vi "CH_LM App DAQ Dispatcher.vi"(4 "DAQ Command":T2={"Wait at Rendesvouz"=FALSE, "Command"="", "Sample Collection"=enum."Continuous", "Sample Size"=100, "Collection Mode"=enum."Streaming", "T / ms"=1.0, "NofBins"=7, "Point(s)"=1, "Log Data File"=path "", "Log data to File"=FALSE, "Pause"=FALSE, "Meter Index"=0, "Data format"=0, "Delivery Mode"=enum."Last", "Start/Stop Button"=refnum, "Point(s) Array"=[]} {"Point(s) Array" min=1 max=20000; "Point(s)" min=1 max=20000; "Sample Size" min=1}, 5 "Rendezvous":T4, 6 "error in (no error)":errorcluster, 8 "Devices":T1[](array[typedef]) {"Probe Diameter" format="%#.2g"}, 9 "Parent ref":refnum<vi>) -> (0 "error out":errorcluster, 2 "timed out":bool)   [LabVIEW 2012, in "CH_LM App.lvlib"]
doc: "This VI is used to dispatch new DAQ threads."
uses:
  CH_LM App.lvlib
  _CH_LM/CH_LM FGV Functions.ctl
  CH_LM.lvlib
  CH_LM App DAQ Command.ctl
  CH_LM App DeviceListElement.ctl
  CH_LM/CH_LM Measurement Delivery Mode.ctl
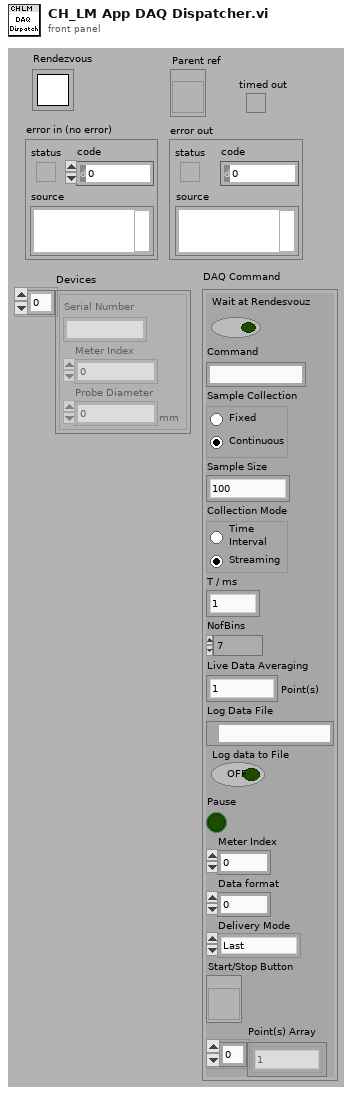
[diagram p1: front panel]
types:
  T1 = typedef "CH_LM App.lvlib/CH_LM App DeviceListElement.ctl" = cluster{"Serial Number":string, "Meter Index":i32, "Probe Diameter":dbl[unit]}
  T2 = typedef "CH_LM App.lvlib/CH_LM App DAQ Command.ctl" = cluster{"Wait at Rendesvouz":bool, "Command":string, "Sample Collection":enum32{"Fixed", "Continuous"}, "Sample Size":i32, "Collection Mode":enum32{"Time\nInterval", "Streaming"}, "T / ms":dbl, "NofBins":i32, "Point(s)":u32, "Log Data File":path, "Log data to File":bool, "Pause":bool, "Meter Index":i32, "Data format":u16, "Delivery Mode":T3, "Start/Stop Button":refnum<vi>, "Point(s) Array":u32[]}
  T3 = typedef "CH_LM.lvlib/CH_LM Measurement Delivery Mode.ctl" = enum16{"Last", "Stream"}
  T4 = typedef "Rendezvous RefNum" = refnum<k1>
  T5 = typedef "CH_LM.lvlib/CH_LM FGV Functions.ctl" = enum16{"create", "get", "set", "remove", "clear", "getBySerial"}
  T6 = enum32{"Invalid", "Standard", "Closed", "Hidden", "Minimized", "Maximized"}
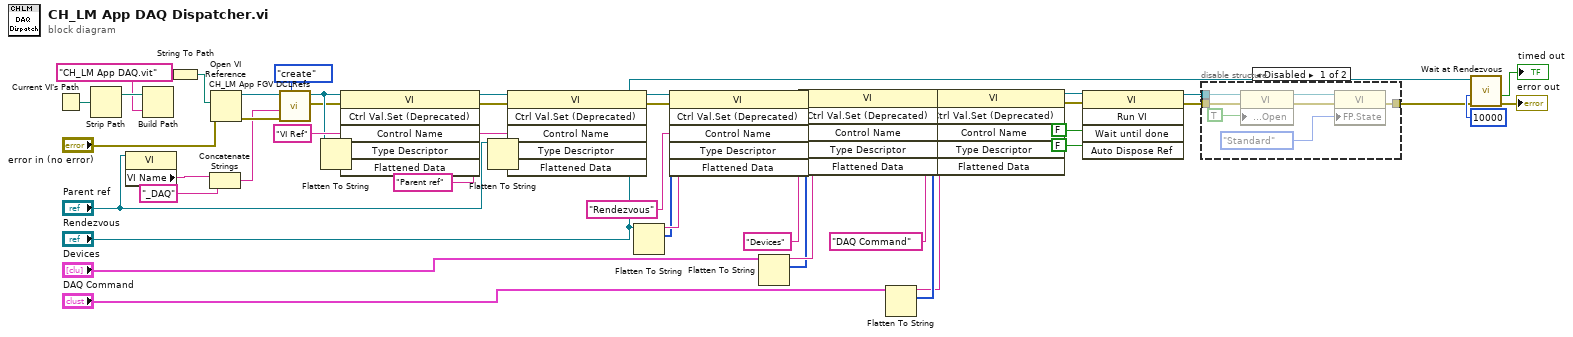
[diagram p0: block diagram]
diagram:
  w2 = "CH_LM App DAQ.vit"
  n1 = Current VI's Path() -> (path=w50:path)
  n2 = Strip Path(path=w50) -> (stripped path=w49:path)  [unwired: 1 out]
  n3 = property class="VI"(reference="Parent ref") -> ("VI Name"=w11:string)  [unwired: 1 in, 2 out]
  n4 = Build Path(base path=w49, name or relative path=w2) -> ()  [unwired: 1 out]
  n5 = String To Path(string=w2) -> (path=w3:path)
  n6 = Concatenate Strings(w11, "_DAQ" ("string")) -> (w9:string)
  n7 = Open VI Reference(vi path=w3, error in (no error)="error in (no error)") -> (vi reference=w34:refnum<vi>, error out=w33:errorcluster)  [unwired: 4 out]
  n8 = call "CH_LM App FGV DCLRefs.vi"("Function"=CH_LM_FGV_Functions."create", "error in (no error)"=w33, "VI Name"=w9, "VI Ref"=w34) -> ("error out"=w30:errorcluster, "VI Ref"=w31:refnum<vi>)  [unwired: 6 out]
  n9 = Flatten To String(anything=w31) -> (data string=w44:string, type string=w45:i16[])  [unwired: 1 in, 3 out]
  n10 = invoke class="VI" method="Ctrl Val.Set (Deprecated)"(reference=w31, error in=w30, "Control Name"="VI Ref", "Type Descriptor"=w45, "Flattened Data"=w44) -> (reference out=w26:refnum<vi>, error out=w23:errorcluster)  [unwired: 1 in, 4 out]
  n11 = Flatten To String(anything="Parent ref") -> (data string=w29:string, type string=w28:i16[])  [unwired: 1 in, 3 out]
  n12 = invoke class="VI" method="Ctrl Val.Set (Deprecated)"(reference=w26, error in=w23, "Control Name"="Parent ref", "Type Descriptor"=w28, "Flattened Data"=w29) -> (reference out=w25:refnum<vi>, error out=w24:errorcluster)  [unwired: 1 in, 4 out]
  n13 = Flatten To String(anything="Rendezvous") -> (data string=w41:string, type string=w40:i16[])  [unwired: 1 in, 3 out]
  n14 = invoke class="VI" method="Ctrl Val.Set (Deprecated)"(reference=w25, error in=w24, "Control Name"="Rendezvous", "Type Descriptor"=w40, "Flattened Data"=w41) -> (reference out=w14:refnum<vi>, error out=w13:errorcluster)  [unwired: 1 in, 4 out]
  n15 = Flatten To String(anything="Devices") -> (data string=w37:string, type string=w36:i16[])  [unwired: 1 in, 3 out]
  n16 = invoke class="VI" method="Ctrl Val.Set (Deprecated)"(reference=w14, error in=w13, "Control Name"="Devices", "Type Descriptor"=w36, "Flattened Data"=w37) -> (reference out=w20:refnum<vi>, error out=w19:errorcluster)  [unwired: 1 in, 4 out]
  n17 = Flatten To String(anything="DAQ Command") -> (data string=w21:string, type string=w22:i16[])  [unwired: 1 in, 3 out]
  n18 = invoke class="VI" method="Ctrl Val.Set (Deprecated)"(reference=w20, error in=w19, "Control Name"="DAQ Command", "Type Descriptor"=w22, "Flattened Data"=w21) -> (reference out=w18:refnum<vi>, error out=w17:errorcluster)  [unwired: 1 in, 4 out]
  n19 = invoke class="VI" method="Run VI"(reference=w18, error in=w17, "Wait until done"=FALSE, "Auto Dispose Ref"=FALSE) -> (reference out=w43:refnum<vi>, error out=w42:errorcluster)  [unwired: 1 in, 3 out]
  n20 = disable-structure shown="Disabled" {
    disable-tunnel: w43 -> [w57 _]
    disable-tunnel: w42 -> [w56 w58]
    disable-tunnel: [w52 w58] -> w1
    frame Disabled {
      n21 = property class="VI"(reference=w57, error in=w56, "Front Panel Window:Open"=TRUE) -> (reference out=w54:refnum<vi>, error out=w53:errorcluster)
      n22 = property class="VI"(reference=w54, error in=w53, "FP.State"=T6."Standard" ("Front Panel Window:State")) -> (error out=w52:errorcluster)  [unwired: 1 out]
    }
    frame Enabled {
    }
  }
  n23 = call <vilib>:"Wait at Rendezvous.vi"("error in (no error)"=w1, "ms timeout (-1)"=10000, "rendezvous"="Rendezvous") -> ("error out"=→"error out":errorcluster, "timed out"=→"timed out":bool)  [unwired: 3 out]
